vi "TEST - Find VI with Focus.vi"(8 "error in (no error)":errorcluster) -> (0 "error out":errorcluster, 2 "pass":bool)   [LabVIEW 2009]
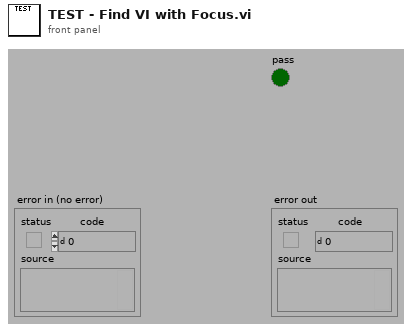
[diagram p1: front panel]
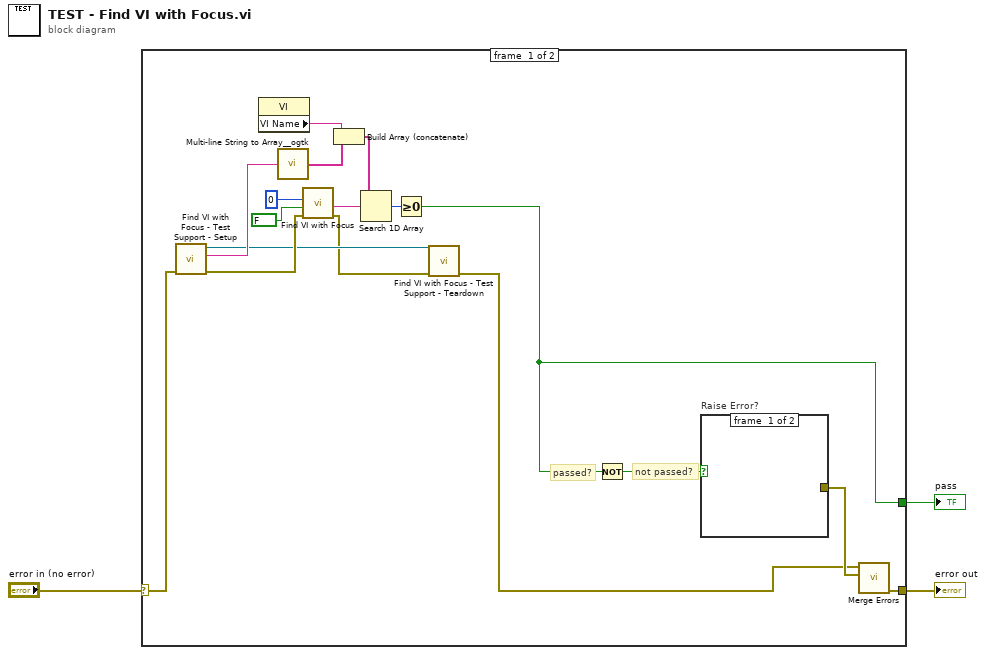
[diagram p0: block diagram]
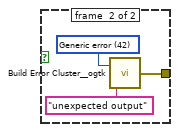
[diagram p2: hidden frame]
diagram:
  n1 = case shown="No Error" "error in (no error)" {
    selector: "error in (no error)" -> [w9 w24]
    tunnel: [w15 _] -> w3
    tunnel: [w20 w24] -> w1
    frame #0 {
      # "not passed?"
      # "passed?"
      n2 = call "Find VI with Focus - Test Support - Setup.vi"("error in (no error)"=w9) -> ("error out"=w8:errorcluster, "VI Name"=w7:string, "VI Renum"=w6:refnum<vi>)  [unwired: 8 in]
      n3 = property class="VI"() -> ("VI Name"=w14:string)  [unwired: 2 in, 2 out]
      n4 = call <userlib>:"Multi-line String to Array__ogtk.vi"("string"=w7) -> ("lines"=w13:string[])
      n5 = call "Find VI with Focus.vi"("error in"=w8, "Exclude Callers"=FALSE, "Exclude Levels"=0) -> ("error out"=w5:errorcluster, "VI Name"=w17:string)  [unwired: 4 in, 3 out]
      n6 = Build Array (concatenate)(w14, w13) -> (w12:string[])
      n7 = Search 1D Array(1D array=w12, element=w17) -> (index of element=w16:i32)  [unwired: 1 in]
      n8 = Greater Or Equal To 0?(x=w16) -> (x >= 0?=w15:bool)
      n9 = call "Find VI with Focus - Test Support - Teardown.vi"("error in (no error)"=w5, "VI Renum"=w6) -> ("error out"=w4:errorcluster)  [unwired: 9 in]
      n10 = Not(x=w15) -> (.not. x?=w18:bool)
      n11 = case "Raise Error?" shown="True" w18 {
        tunnel: [_ w21] -> w19
        frame #0 {
        }
        frame #1 {
          w22 = 42 items=["No error", "Argument error", "Memory is full", "Out of zone", "End of file", "File already open", "Generic file I/O error", "File not found", "File permission error", "Disk is full", "Duplicate path", "Too many files open", "System feature not enabled", "Resource file not found", "Cannot add resource", "Resource not found", "Image not found", "Image memory error", "Pen does not exist", "Config type invalid", "Config token not found", "Config parse error", "Config memory error", "Bad external code format", "Bad external code offset", "External code not present", "Null window", "Destroy window error", "Null menu", "Print aborted", "Bad print record", "Print driver error", "Windows error during printing", "Memory error during printing", "Print dialog error", "Generic print error", "Invalid device refnum", "Device not found", "Device parameter error", "Device unit error", "Cannot open device", "Device call aborted", "Generic error", "Cancelled by user", "Object ID too low", "Object ID too high", "Object not in heap", "Unknown heap", "Unknown object (invalid DefProc)", "Unknown object (DefProc not in table)", "Message out of range", "Invalid (null) method", "Unknown message", "Manager call not supported", "Bad address", "Network operation in progress", "Network operation timed out", "Connection is busy", "Network attribute not supported", "Network error", "Address in use", "System out of memory", "Connection aborted", "Connection refused", "Not connected", "Already connected", "Connection closed", "Initialization error (interapplication manager)", "Bad occurrence", "Wait on unbound occurrence handler", "Occurrence queue overflow", "Datalog type conflict", "Unused", "Unrecognized type (interapplication manager)", "Memory corrupt", "Failed to make temporary DLL", "Old CIN version", "Drag socket not found", "Failed to load drop-object", "Failed to register OLE object", "Failed to release OLE object", "Format specifier type mismatch", "Unknown format specifier", "Too few format specifiers", "Too many format specifiers", "Scan failed", "Newer CIN version", "Error converting to variant", "Runtime menu error", "Password tampered", "Variant attribute not found", "Incompatible variant data type", "Event data is not available", "Event Store is not present", "Occurrence is not found", "Event Queue is not created", "Event info is not available", "Refnum passed is NULL", "Error retrieving Class GUID", "Error retrieving CoClass GUID", "Error retrieving TypeLib GUID.", "Bad built application magic bytes.", "Specific driver is different from the specific driver associated with the Logical Name.", "There is no session opened to the class driver.", "Max Error", "MAX - Error with config objects", "MAX - Error loading configuration", "MAX - Group not supported"]
          n12 = call <userlib>:"Build Error Cluster__ogtk.vi"("String to Prepend to source (\"\")"="unexpected output" ("String to Prepend to source (\"\")"), "code"=w22) -> ("error out"=w21:errorcluster)
        }
      }
      n13 = call <vilib>:"Merge Errors.vi"("error in 2 (no error)"=w19, "error in 1 (no error)"=w4) -> ("error out"=w20:errorcluster)  [unwired: 5 in]
    }
    frame #1 {
    }
  }
  "pass" <- w3
  "error out" <- w1
